vi "Untitled 1.vi"() -> ()   [LabVIEW 2017]
uses:
  <vilib>/Utility/miscctls.llb/LVRowAndColumnTypeDef.ctl
panel:
  in  "Autosizing Columns?":bool
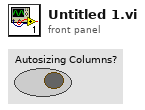
[diagram p1: front panel]
types:
  T1 = typedef "LVRowAndColumnTypeDef.ctl" = cluster{"Row":i32, "Column":i32}
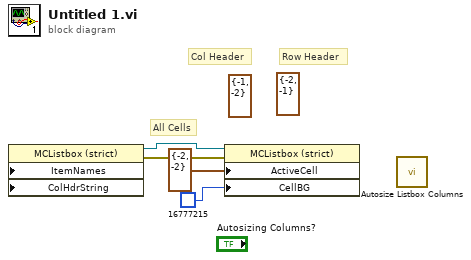
[diagram p0: block diagram]
diagram:
  (unwired) T1 {"Row"=-2, "Column"=-1} ("Active Cell:Active Cell")
  (unwired) T1 {"Row"=-1, "Column"=-2} ("Active Cell:Active Cell")
  # "Row Header"
  # "Col Header"
  # "All Cells"
  n1 = property class="MCListbox (strict)" props=["ItemNames", "ColHdrString"]() -> (reference out=w2:refnum<vi>, error out=w1:errorcluster)  [unwired: 4 in]
  n2 = property class="MCListbox (strict)"(reference=w2, error in=w1, "ActiveCell"=T1 {"Row"=-2, "Column"=-2} ("Active Cell:Active Cell"), "CellBG"=u32 16777215) -> ()  [unwired: 2 out]
  n3 = call "Autosize Listbox Columns.vi"() -> ()  [unwired: 7 in, 1 out]
